vi "Config AO Wav.vi"(6 "Channel config":T1={"Frequency"=10.0, "Voltage"=1.0, "Signal type"=enum."Sine Wave", "Square wave duty cycle (%)"=50.0, "physical channels"="", "name to assign"="", "Phase"=1.0} {"Square wave duty cycle (%)" format="%0.2f"}, 7 "Sampling info":cluster{"Fs":dbl, "#s":dbl}={"Fs"=1000.0, "#s"=1000.0} {"Fs" format="%.2p"}, 8 "error in":errorcluster, 11 "task in":refnum<k21>) -> (0 "error out":errorcluster, 3 "task out":refnum<k21>, 4 "AO Waveform Graph":waveform(dbl)(graph))   [LabVIEW 2019]
doc: "This example demonstrates how to acquire a continuous amount of data (Waveform) using the DAQ device's internal clock. It also shows how to synchronize two devices for different device families (E Series, S Series, M Series, X Series, DSA, and SC Express), to simultaneously acquire the data.\n\nFor instructions on how to connect your signals to the DAQ device, refer to your device documentation."
uses:
  <vilib>/DAQmx/write.llb/DAQmx Write (Analog Wfm 1Chan NSamp).vi
  <vilib>/DAQmx/create/channels.llb/DAQmx Create Channel (AO-Voltage-Basic).vi
  <vilib>/DAQmx/configure/timing.llb/DAQmx Timing (Sample Clock).vi
  <vilib>/DAQmx/miscellaneous.llb/DAQmx Fill In Error Info.vi
  <vilib>/measure/NI_MABase.lvlib
panel:
  # "Config AO - Waveform"
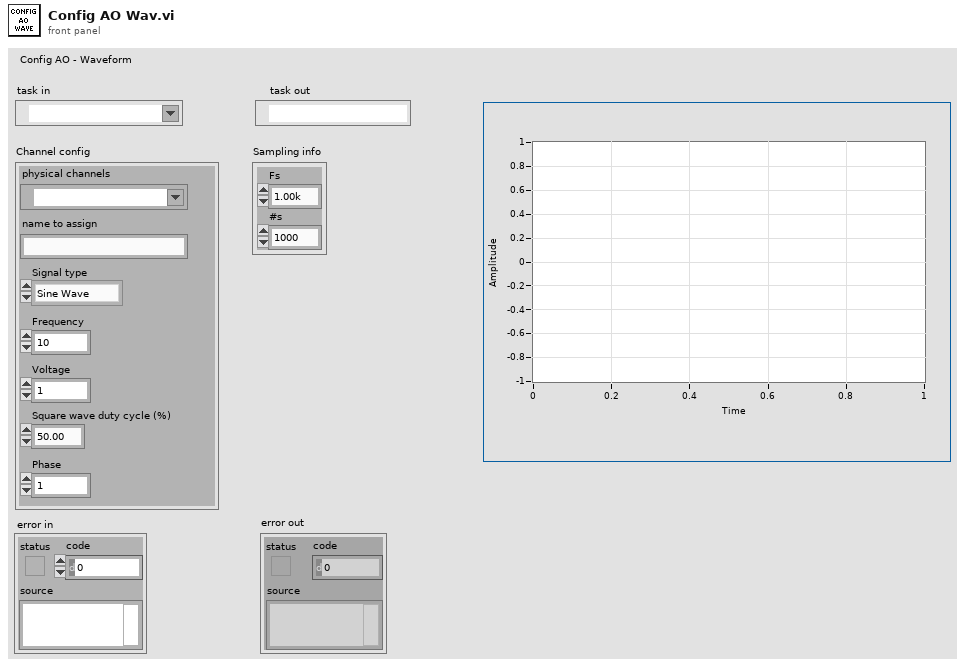
[diagram p1: front panel]
types:
  T1 = cluster{"Frequency":dbl, "Voltage":dbl, "Signal type":enum16{"Sine Wave", "Triangle Wave", "Square Wave", "Sawtooth Wave"}, "Square wave duty cycle (%)":dbl, "physical channels":tag, "name to assign":string, "Phase":dbl}
  T2 = enum16{"Sine Wave", "Triangle Wave", "Square Wave", "Sawtooth Wave"}
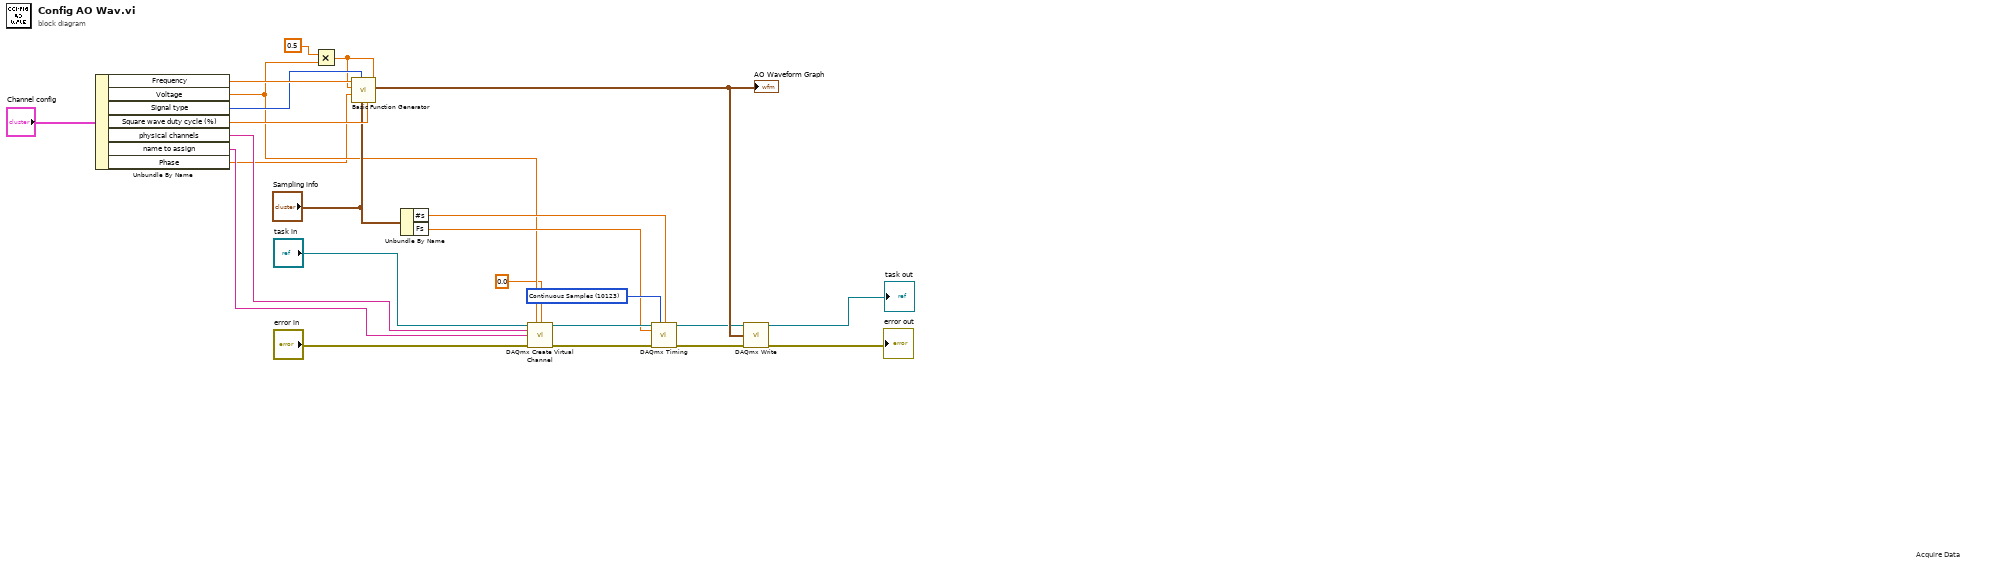
[diagram p0: block diagram]
diagram:
  w10 = 10123 items=["Finite Samples"=10178, "Continuous Samples"=10123, "Hardware Timed Single Point"=12522] ("sample mode")
  # "Acquire Data"
  n1 = Unbundle By Name("Channel config") -> ("Frequency"=w18:dbl, "Voltage"=w5:dbl, "Signal type"=w16:T2, "Square wave duty cycle (%)"=w17:dbl, "physical channels"=w3:tag, "name to assign"=w2:string, "Phase"=w1:dbl)
  n2 = Multiply(x=0.5, y=w5) -> (x*y=w6:dbl)
  n3 = call <vilib>:"Basic Function Generator.vi"("offset"=w6, "square wave duty cycle (%)"=w17, "sampling info"="Sampling info", "signal type"=w16, "phase"=w1, "amplitude"=w6, "frequency"=w18) -> ("signal out"=w24:waveform(dbl))  [unwired: 2 in, 2 out]
  "AO Waveform Graph" <- w24
  n4 = Unbundle By Name("Sampling info") -> ("#s"=w9:dbl, "Fs"=w8:dbl)
  n5 = call-poly <vilib>:"DAQmx Create Virtual Channel.vi"("task in"="task in", "maximum value"=w5, "minimum value"=0.0, "physical channels"=w3, "name to assign"=w2, "error in"="error in") -> ("task out"=w15:refnum<k21>, "error out"=w14:errorcluster)  [unwired: 8 in]
  n6 = call-poly <vilib>:"DAQmx Timing.vi"("task/channels in"=w15, "sample mode"=w10, "samples per channel"=w9, "rate"=w8, "error in"=w14) -> ("task out"=w12:refnum<k21>, "error out"=w13:errorcluster)  [unwired: 9 in]
  n7 = call-poly <vilib>:"DAQmx Write.vi"("task/channels in"=w12, "data"=w24, "error in"=w13) -> ("task out"=→"task out":refnum<k21>, "error out"=→"error out":errorcluster)  [unwired: 10 in, 1 out]
